vi "GetTimeElapsed.vi"(11 "Start Time (sec)":dbl) -> (3 "Time Elapsed (sec)":dbl)   [LabVIEW 2012, in "LV-Utilities.lvlib"]
doc: "This VI gets the time elasped in seconds since a specific start time."
uses:
  LV-Utilities.lvlib
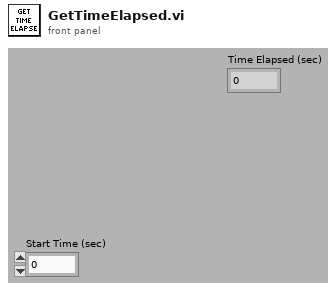
[diagram p1: front panel]
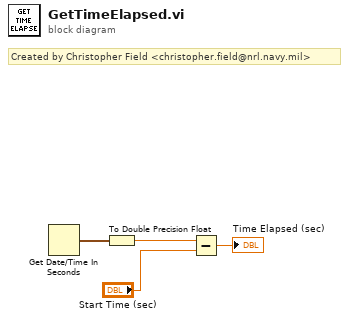
[diagram p0: block diagram]
diagram:
  # "Created by Christopher Field <christopher.field@nrl.navy.mil>"
  n1 = Get Date/Time In Seconds() -> (seconds since 1Jan1904=w4:timestamp)
  n2 = To Double Precision Float(number=w4) -> (double precision float=w3:dbl)
  n3 = Subtract(x=w3, y="Start Time (sec)") -> (x-y=→"Time Elapsed (sec)":dbl)
